vi "Home All.vi"(0 "Notifier Name":string, 11 "Error In":errorcluster) -> (4 "Notifier Name Dup":string, 6 "Dichroic Pos":i32, 8 "Filter Wheel Pos":i32, 10 "Disk Pos":i32, 13 "Error":bool, 15 "Error Out":errorcluster)   [LabVIEW 2020]
uses:
  Spinning Disk Type Defs/SD Notifer Data.ctl
  Spinning Disk Type Defs/SD Actions.ctl
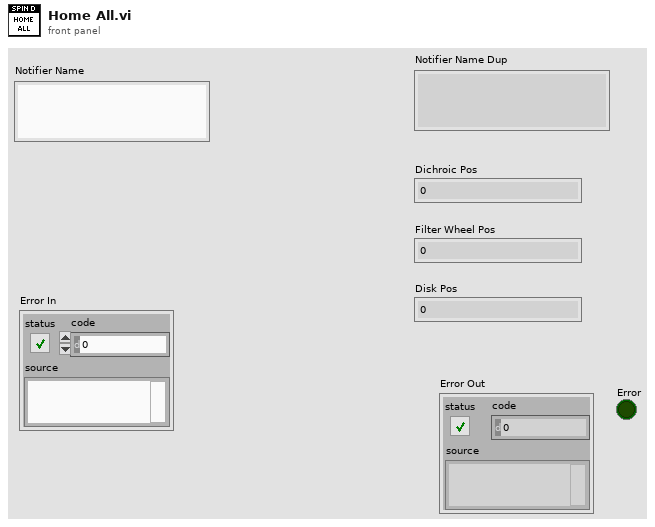
[diagram p1: front panel]
types:
  T1 = typedef "SD Notifer Data.ctl" = cluster{"Actions":T2, "Disk On?":bool, "Dichroic Pos.":i32, "Filter Wheel Pos.":i32, "Disk Pos.":i32, "Recived":bool, "Num Pos":i32[]}
  T2 = typedef "SD Actions.ctl" = enum16{"Status", "Get All Pos.", "Get Num. Pos.", "Home All", "Set Filter Wheel Pos.", "Set Disk Pos.", "Set Dichroic Pos.", "Disk On", "Disk Off", "Quit"}
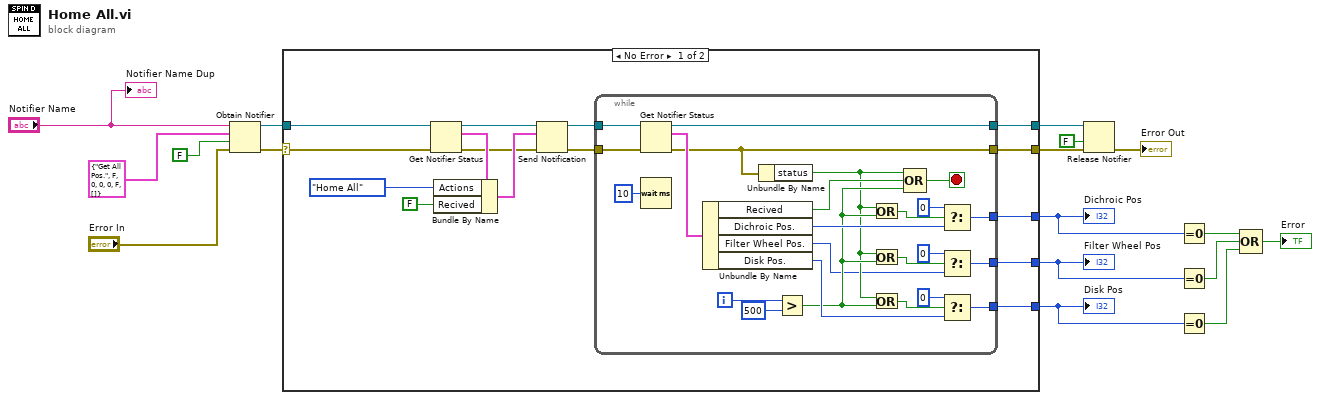
[diagram p0: block diagram]
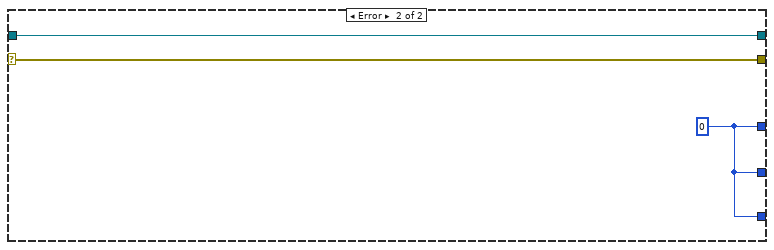
[diagram p2: hidden frame]
diagram:
  n1 = Obtain Notifier(name (unnamed)="Notifier Name", notification data type=T1 {"Actions"=enum."Get All Pos.", "Disk On?"=FALSE, "Dichroic Pos."=0, "Filter Wheel Pos."=0, "Disk Pos."=0, "Recived"=FALSE, "Num Pos"=[]} ("XLight Notifier Data"), create if not found? (T)=FALSE, error in (no error)="Error In") -> (notifier out=w13:refnum<notifier>, error out=w10:errorcluster)  [unwired: 1 out]
  n2 = case shown="No Error" w10 {
    selector: w10 -> [w31 w58]
    tunnel: w13 -> [w32 w59]
    tunnel: [w21 w59] -> w12
    tunnel: [w22 w58] -> w9
    tunnel: [w20 w57] -> w7
    tunnel: [w19 w57] -> w5
    tunnel: [w18 w57] -> w6
    frame No Error {
      n3 = Get Notifier Status(notifier=w32, error in (no error)=w31) -> (notifier out=w27:refnum<notifier>, current notification=w30:T1, error out=w25:errorcluster)  [unwired: 2 out]
      n4 = Bundle By Name(cluster=w30, "Actions"=SD_Actions."Home All", "Recived"=FALSE) -> (w26:T1)
      n5 = Send Notification(notification=w26, notifier=w27, error in (no error)=w25) -> (notifier out=w24:refnum<notifier>, error out=w23:errorcluster)
      n6 = while {
        tunnel: w24 -> [w54]
        tunnel: w23 -> [w53]
        tunnel: [w46] -> w22
        tunnel: [w45] -> w21
        tunnel: [w44] -> w20
        tunnel: [w34] -> w19
        tunnel: [w33] -> w18
        i -> [w56]
        stop <- w47 stop-if-true
        n7 = Get Notifier Status(notifier=w54, error in (no error)=w53) -> (notifier out=w45:refnum<notifier>, current notification=w52:T1, error out=w46:errorcluster)  [unwired: 2 out]
        n8 = Wait (ms)(milliseconds to wait=u32 10) -> ()  [unwired: 1 out]
        n9 = Unbundle By Name(w52) -> ("Recived"=w51:bool, "Dichroic Pos."=w50:i32, "Filter Wheel Pos."=w35:i32, "Disk Pos."=w38:i32)
        n10 = Unbundle By Name(w46) -> ("status"=w36:bool)
        n11 = Greater?(x=w56, y=500) -> (0:w37:bool)
        n12 = Or(x=w36, y=w37) -> (x .or. y?=w48:bool)
        n13 = Or(x=w36, y=w37) -> (x .or. y?=w42:bool)
        n14 = Or(x=w36, y=w37) -> (x .or. y?=w39:bool)
        n15 = Compound Arithmetic op=OR(w36, w51, w37) -> (w47:bool)
        n16 = Select(t=0, s=w48, f=w50) -> (s? t:f=w44:i32)
        n17 = Select(t=0, s=w42, f=w35) -> (s? t:f=w34:i32)
        n18 = Select(t=0, s=w39, f=w38) -> (s? t:f=w33:i32)
      }
    }
    frame Error {
      w57 = 0 ("Filter Wheel Pos.")
    }
  }
  "Dichroic Pos" <- w7
  "Filter Wheel Pos" <- w5
  "Disk Pos" <- w6
  n19 = Release Notifier(notifier=w12, force destroy? (F)=FALSE, error in (no error)=w9) -> (error out=→"Error Out":errorcluster)  [unwired: 2 out]
  n20 = Equal To 0?(x=w7) -> (x = 0?=w4:bool)
  n21 = Equal To 0?(x=w5) -> (x = 0?=w3:bool)
  n22 = Equal To 0?(x=w6) -> (x = 0?=w2:bool)
  n23 = Compound Arithmetic op=OR(w4, w3, w2) -> (→"Error":bool)
  "Notifier Name Dup" <- "Notifier Name"
